vi "set_amplitude.vi"(8 "error in (no error)":errorcluster, 10 "Amplitude (Vpp)":dbl, 11 "Keysight 33511B in":refnum<class "Keysight 33511B.lvclass">) -> (0 "error out":errorcluster, 3 "Keysight 33511B out":refnum<class "Keysight 33511B.lvclass">)   [LabVIEW 2020, in "Keysight 33511B.lvclass"]
uses:
  Keysight 33511B.lvclass
  Keysight 33511B.lvclass/Keysight 33511B.ctl
  Function Generator/Function Generator.lvclass
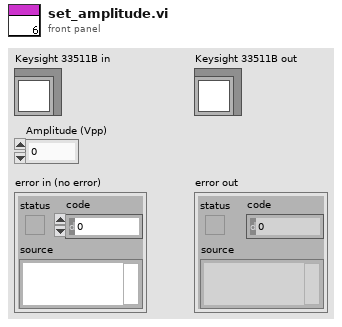
[diagram p1: front panel]
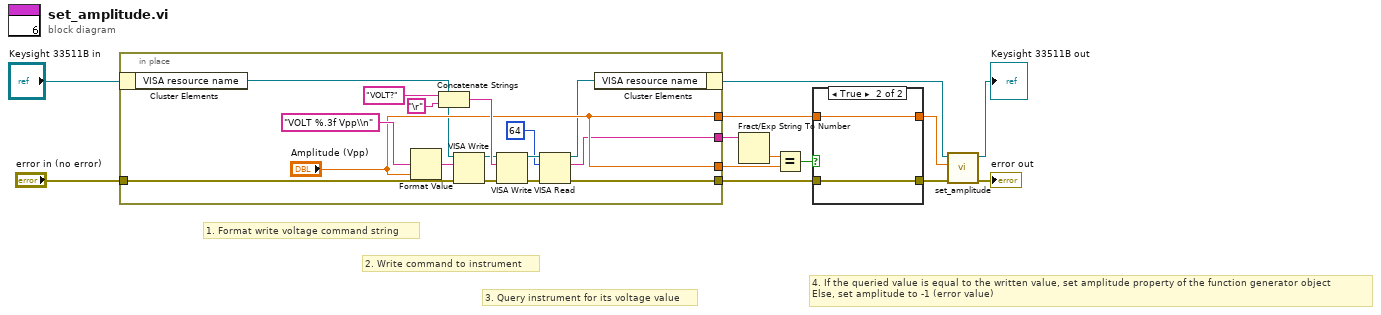
[diagram p0: block diagram]
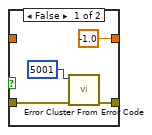
[diagram p2: hidden frame]
diagram:
  # "4. If the queried value is equal to the written value, set amplitude property of the function generator object\nElse, set amplitude to -1 (error value)"
  # "3. Query instrument for its voltage value"
  # "2. Write command to instrument"
  # "1. Format write voltage command string"
  n1 = in-place {
    in-place-border: "error in (no error)" -> [w19]
    in-place-border: ["Amplitude (Vpp)"] -> w7
    in-place-border: [w18] -> w6
    in-place-border: ["Amplitude (Vpp)"] -> w5
    in-place-border: [w16] -> w4
    n2 = in-place-cluster #1("Keysight 33511B in") -> ("VISA resource name"=w14:refnum<visa-resource-name>)
    n3 = Format Value(format string="VOLT %.3f Vpp\\n", value (0)="Amplitude (Vpp)") -> (output string=w24:string)  [unwired: 1 in]
    n4 = Concatenate Strings("VOLT?", "\r") -> (w27:string)
    n5 = VISA Write(VISA resource name=w14, write buffer=w24, error in (no error)=w19) -> (VISA resource name out=w25:refnum<visa-resource-name>, error out=w26:errorcluster)  [unwired: 1 out]
    n6 = VISA Write(VISA resource name=w25, write buffer=w27, error in (no error)=w26) -> (VISA resource name out=w28:refnum<visa-resource-name>, error out=w29:errorcluster)  [unwired: 1 out]
    n7 = VISA Read(VISA resource name=w28, byte count=u32 64, error in (no error)=w29) -> (VISA resource name out=w15:refnum<visa-resource-name>, read buffer=w16:string, error out=w18:errorcluster)  [unwired: 1 out]
    n8 = in-place-cluster #1("VISA resource name"=w15) -> (w1:refnum<class "Keysight 33511B.lvclass">)
  }
  n9 = Fract/Exp String To Number(string=w4) -> (number=w11:dbl)  [unwired: 3 in, 1 out]
  n10 = Equal?(x=w11, y=w5) -> (x = y?=w10:bool)
  n11 = case shown="True" w10 {
    tunnel: w7 -> [_ w35]
    tunnel: w6 -> [w31 w34]
    tunnel: [-1.0 w35] -> w8
    tunnel: [w30 w34] -> w9
    frame False {
      n12 = call <vilib>:"Error Cluster From Error Code.vi"("error in (no error)"=w31, "error code (0)"=5001) -> ("error out"=w30:errorcluster)  [unwired: 7 in]
    }
    frame True {
    }
  }
  n13 = call-parent "set_amplitude.vi"("error in (no error)"=w9, "Amplitude"=w8, "Function Generator in"=w1) -> ("error out"=→"error out":errorcluster, "Function Generator out"=→"Keysight 33511B out":refnum<class "Keysight 33511B.lvclass">)  [unwired: 7 in]
